vi "获取particle中心坐标.vi"(11 "数组输入":dbl[][](array[numeric])) -> (3 "数组输出":cluster{"Numeric":dbl, "Numeric":dbl}[](array[cluster]))   [LabVIEW 2014]
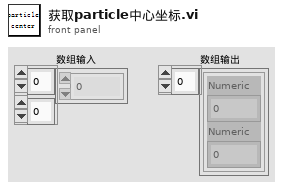
[diagram p1: front panel]
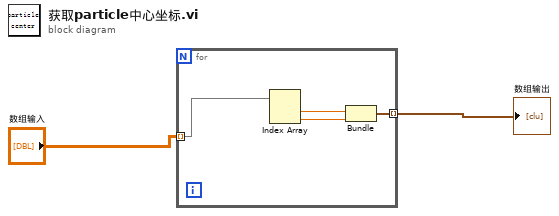
[diagram p0: block diagram]
diagram:
  n1 = for {
    tunnel: "数组输入" -> [w6] mode=indexing
    tunnel: [w3] -> w2 mode=indexing
    n2 = Index Array(array=w6) -> (element #1=w5:dbl, element #2=w4:dbl)  [unwired: 2 in]
    n3 = Bundle("Numeric"=w5, "Numeric"=w4) -> (w3:cluster{"Numeric":dbl, "Numeric":dbl})  [unwired: 1 in]
  }
  "数组输出" <- w2
